vi "Execute.vi"(8 "error in (no error)":errorcluster, 11 "TAS_Message in":refnum<class "TAS_Message.lvclass">) -> (0 "error out":errorcluster, 3 "TAS_Message out":refnum<class "TAS_Message.lvclass">)   [LabVIEW 2012, in "TAS_Message.lvclass"]
uses:
  TAS_Message.lvclass
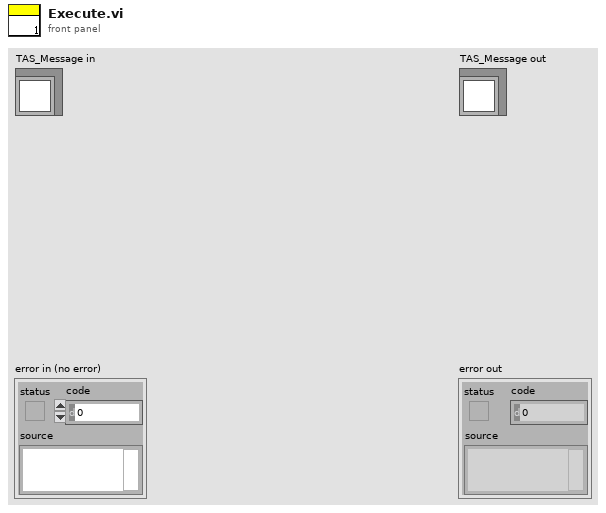
[diagram p1: front panel]
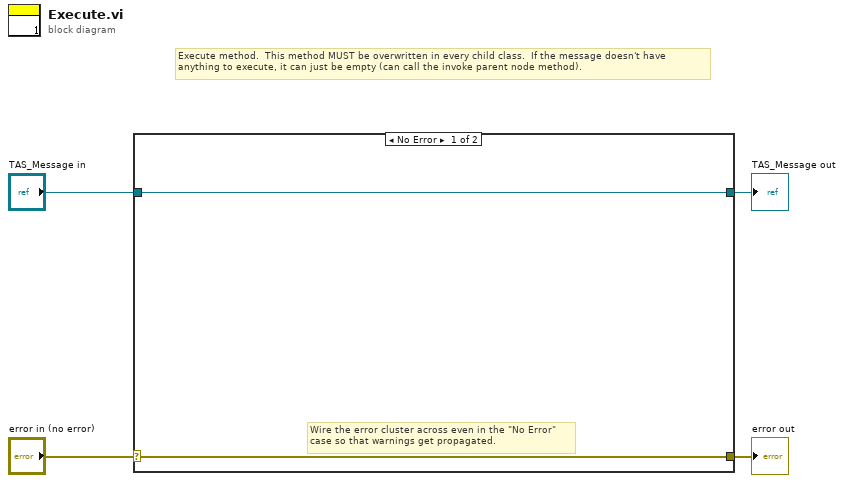
[diagram p0: block diagram]
diagram:
  # "Execute method.  This method MUST be overwritten in every child class.  If the message doesn't have\nanything to execute, it can just be empty (can call the invoke parent node method)."
  n1 = case shown="No Error" "error in (no error)" {
    selector: "error in (no error)" -> [w5 w8]
    tunnel: [w5 w8] -> w3
    tunnel: [w6 w7] -> w1
    tunnel: "TAS_Message in" -> [w6 w7]
    frame No Error {
      # "Wire the error cluster across even in the \"No Error\"\ncase so that warnings get propagated."
    }
    frame Error {
    }
  }
  "error out" <- w3
  "TAS_Message out" <- w1
